vi "Set Name at Path Array.vi"(0 "Variant in":variant, 2 "Path in":string[](array[string]), 7 "Name":string, 11 "error in (no error)":errorcluster) -> (4 "Variant out":variant, 15 "error out":errorcluster)   [LabVIEW 2017, in "Advanced Variant Tools.lvlib"]
uses:
  Advanced Variant Tools.lvlib
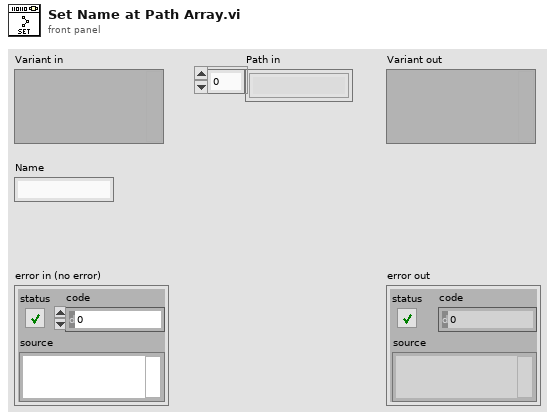
[diagram p1: front panel]
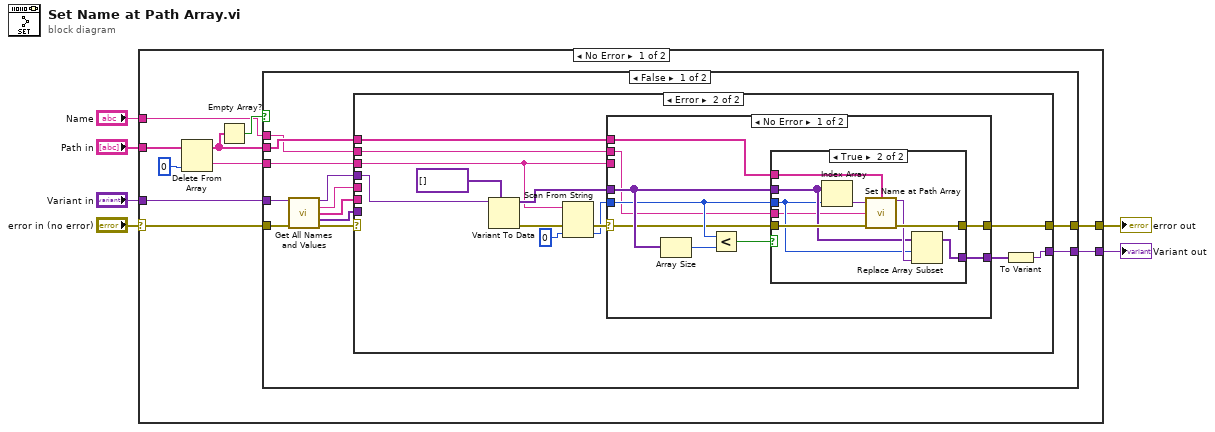
[diagram p0: block diagram]
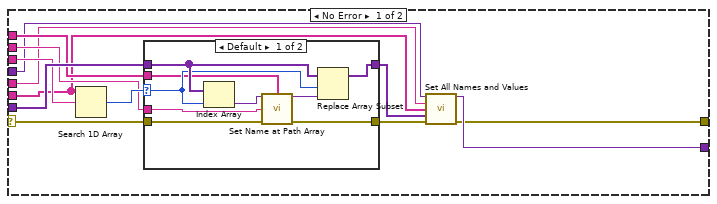
[diagram p2: hidden frame]
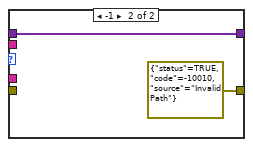
[diagram p3: hidden frame]
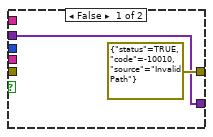
[diagram p4: hidden frame]
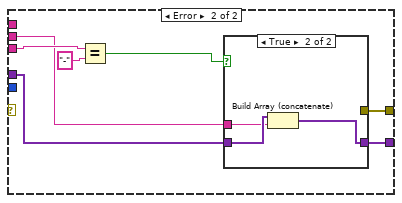
[diagram p5: hidden frame]
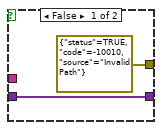
[diagram p6: hidden frame]
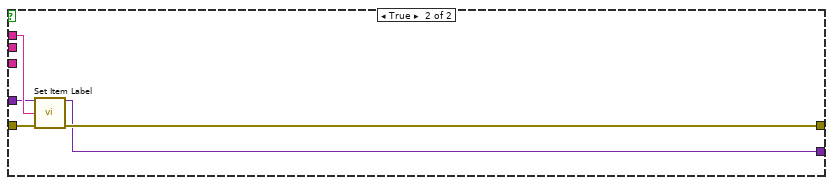
[diagram p7: hidden frame]
diagram:
  n1 = case shown="No Error" "error in (no error)" {
    selector: "error in (no error)" -> [w15 w104]
    tunnel: "Path in" -> [w12 _]
    tunnel: "Variant in" -> [w16 w103]
    tunnel: [w8 w104] -> w4
    tunnel: [w9 w103] -> w2
    tunnel: "Name" -> [w10 _]
    frame No Error {
      n2 = Delete From Array(array=w12, index=0) -> (deleted portion=w14:string, array with subset deleted=w7:string[])  [unwired: 1 in]
      n3 = Empty Array?(array=w7) -> (empty?=w11:bool)
      n4 = case shown="False" w11 {
        tunnel: w16 -> [w28 w98]
        tunnel: w15 -> [w27 w102]
        tunnel: w14 -> [w24 _]
        tunnel: w7 -> [w23 _]
        tunnel: w10 -> [w22 w99]
        tunnel: [w18 w100] -> w9
        tunnel: [w17 w101] -> w8
        frame False {
          n5 = call "Get All Names and Values.vi"("Variant (Cluster) In"=w28, "error in"=w27) -> ("Variant (Cluster) Out"=w20:variant, "Name"=w19:string, "Element Names"=w21:string[], "Values"=w25:variant[], "error out"=w26:errorcluster)  [unwired: 9 in]
          n6 = case shown="Error" w26 {
            selector: w26 -> [w39 _]
            tunnel: w20 -> [w29 w62]
            tunnel: w24 -> [w38 w53]
            tunnel: w21 -> [w34 _]
            tunnel: w25 -> [w40 _]
            tunnel: w23 -> [w37 w57]
            tunnel: w22 -> [w36 w58]
            tunnel: w19 -> [w35 _]
            tunnel: [w31 w56] -> w18
            tunnel: [w30 w54] -> w17
            frame No Error {
              n7 = Search 1D Array(1D array=w34, element=w38) -> (index of element=w41:i32)  [unwired: 1 in]
              n8 = case shown="Default" w41 {
                selector: w41 -> [w46 _]
                tunnel: [w48 errorcluster {"status"=TRUE, "code"=-10010, "source"="Invalid Path"} ("error IO")] -> w32
                tunnel: w40 -> [w47 w51]
                tunnel: w39 -> [w49 _]
                tunnel: w37 -> [w43 _]
                tunnel: w36 -> [w42 _]
                tunnel: [w44 w51] -> w33
                frame Default {
                  n9 = Index Array(array=w47, index=w46) -> (element=w50:variant)
                  n10 = call "Set Name at Path Array.vi"("Variant in"=w50, "Path in"=w43, "Name"=w42, "error in (no error)"=w49) -> ("Variant out"=w45:variant, "error out"=w48:errorcluster)  [unwired: 10 in]
                  n11 = Replace Array Subset(array=w47, new element=w45, index=w46) -> (w44:variant[])
                }
                frame -1 {
                }
              }
              n12 = call "Set All Names and Values.vi"("Variant (Cluster) In"=w29, "Name"=w35, "Element Names"=w34, "values"=w33, "error in"=w32) -> ("Variant (Cluster) Out"=w31:variant, "error out"=w30:errorcluster)  [unwired: 9 in]
            }
            frame Error {
              n13 = Variant To Data(type=variant[] [], Variant=w62) -> (data=w60:variant[], error out=w59:errorcluster)  [unwired: 1 in]
              n14 = Scan From String(input string=w53, error in=w59, default 1=0 ("default value 1")) -> (error out=w64:errorcluster, output 1=w63:i32)  [unwired: 2 in, 2 out]
              n15 = case shown="No Error" w64 {
                selector: w64 -> [w68 _]
                tunnel: [w69 w92] -> w54
                tunnel: w63 -> [w72 _]
                tunnel: w60 -> [w73 w88]
                tunnel: [w74 w86] -> w55
                tunnel: w58 -> [w67 w87]
                tunnel: w57 -> [w66 _]
                tunnel: w53 -> [_ w91]
                frame No Error {
                  n16 = Array Size(array=w73) -> (size(s)=w71:i32)
                  n17 = Less?(x=w72, y=w71) -> (x < y?=w70:bool)
                  n18 = case shown="True" w70 {
                    tunnel: [w75 w82] -> w74
                    tunnel: w73 -> [w75 w80]
                    tunnel: w72 -> [_ w79]
                    tunnel: [errorcluster {"status"=TRUE, "code"=-10010, "source"="Invalid Path"} ("error IO") w83] -> w69
                    tunnel: w68 -> [_ w84]
                    tunnel: w67 -> [_ w77]
                    tunnel: w66 -> [_ w78]
                    frame False {
                    }
                    frame True {
                      n19 = Index Array(array=w80, index=w79) -> (element=w85:variant)
                      n20 = call "Set Name at Path Array.vi"("Variant in"=w85, "Path in"=w78, "Name"=w77, "error in (no error)"=w84) -> ("Variant out"=w81:variant, "error out"=w83:errorcluster)  [unwired: 10 in]
                      n21 = Replace Array Subset(array=w80, new element=w81, index=w79) -> (w82:variant[])
                    }
                  }
                }
                frame Error {
                  n22 = Equal?(x=w91, y="-") -> (x = y?=w89:bool)
                  n23 = case shown="True" w89 {
                    tunnel: [errorcluster {"status"=TRUE, "code"=-10010, "source"="Invalid Path"} ("error IO") _] -> w92
                    tunnel: w88 -> [w93 w97]
                    tunnel: w87 -> [_ w96]
                    tunnel: [w93 w95] -> w86
                    frame False {
                    }
                    frame True {
                      n24 = Build Array (concatenate)(w97, w96) -> (w95:variant[])
                    }
                  }
                }
              }
              n25 = To Variant(anything=w55) -> (Variant=w56:variant)
            }
          }
        }
        frame True {
          n26 = call "Set Item Label.vi"("Variant in"=w98, "Name"=w99, "error in (no error)"=w102) -> ("Variant out"=w100:variant, "error out"=w101:errorcluster)  [unwired: 11 in]
        }
      }
    }
    frame Error {
    }
  }
  "error out" <- w4
  "Variant out" <- w2
